vi "Actor Core.vi"(8 "error in":errorcluster, 11 "IMAQdx Actor in":refnum<class "IMAQdx Actor.lvclass">) -> (0 "error out":errorcluster, 3 "Actor out":refnum<class "Actor.lvclass">)   [LabVIEW 2020, in "IMAQdx Actor.lvlib" / "IMAQdx Actor.lvclass"]
doc: "(<B>Filename</B>: Actor Framework.lvlib:Actor.lvclass:Actor Core.vi)\n\nReceives messages to the actor, reacts to them, and initiates any error handling that may shut the actor down.\n\nDescendant classes may override this VI to append parallel tasks for the actor to complete while it handles messages. Overrides use the Call Parent Method node."
uses:
  IMAQdx Actor.lvclass
  C:/Users/AlexK/work/LabVIEW Programme/POLARIS-AS-3-Cams/Submodules/HIJ Vision/Camera Actors/Camera Actor/Camera Actor/Camera Actor.lvclass
  C:/Program Files (x86)/National Instruments/LabVIEW 2020/vi.lib/ActorFramework/Actor/Actor.lvclass
  <vilib>/ActorFramework/Actor/Actor.lvclass
  Camera Actor/Camera Actor/Operation Mode.ctl
  <vilib>/userdefined/High Color/IMAQdx.ctl
  <vilib>/vision/Image Controls.llb/IMAQ Image.ctl
  Camera Actor/Camera Actor/Camera Actor.lvclass/Camera Actor.ctl
  IMAQdx Actor.lvclass/IMAQdx Actor.ctl
  <vilib>/ActorFramework/Actor/Actor.lvclass/Actor.ctl
  <vilib>/ActorFramework/Message Enqueuer/Message Enqueuer.lvclass/Message Enqueuer.ctl
  Camera Actor/Camera Actor Messages/Publish Image Msg/Publish Image Msg.lvclass/Publish Image Msg.ctl
  <vilib>/ActorFramework/Report Error Msg/Report Error Msg.lvclass/Report Error Msg.ctl
  Camera Actor/Camera Actor/Write Image ref.vi
  <vilib>/ActorFramework/Message Enqueuer/Init from Existing Queue.vi
  <vilib>/ActorFramework/Message Enqueuer/Enqueue.vi
  Camera Actor/Camera Actor Messages/Publish Image Msg/Publish Image Msg.lvclass
  C:/Program Files (x86)/National Instruments/LabVIEW 2020/vi.lib/ActorFramework/Message/Message.lvclass
  <vilib>/ActorFramework/Report Error Msg/Report Error Msg.lvclass
  <vilib>/ActorFramework/Message Priority Queue/Priority Enqueue.vi
  Camera Actor/Camera Actor/Camera Actor.lvclass
  <vilib>/ActorFramework/Message Enqueuer/Message Enqueuer.lvclass
  <vilib>/vision/driver/NI_Vision_Acquisition_Software.lvlib
panel:
  in  "Image":T1
  in  "Session In":T2 caption="Session"
  in  "Mode":T3=enum."Stop"
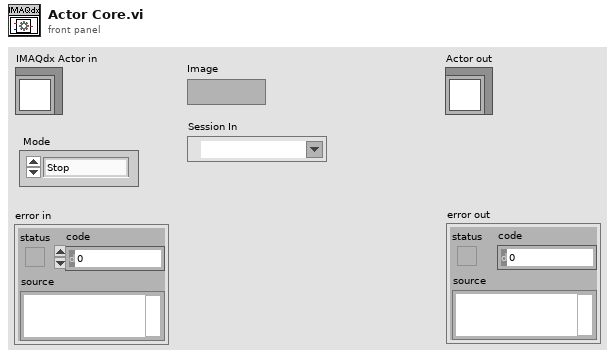
[diagram p1: front panel]
types:
  T1 = typedef "IMAQ Image.ctl" = refnum<image>
  T2 = typedef "IMAQdx.ctl" = refnum<k21>
  T3 = typedef "Camera Actor.lvlib/Camera Actor.lvclass/Operation Mode.ctl" = enum16{"Run", "Stop", "Exit", "Error", "Restart"}
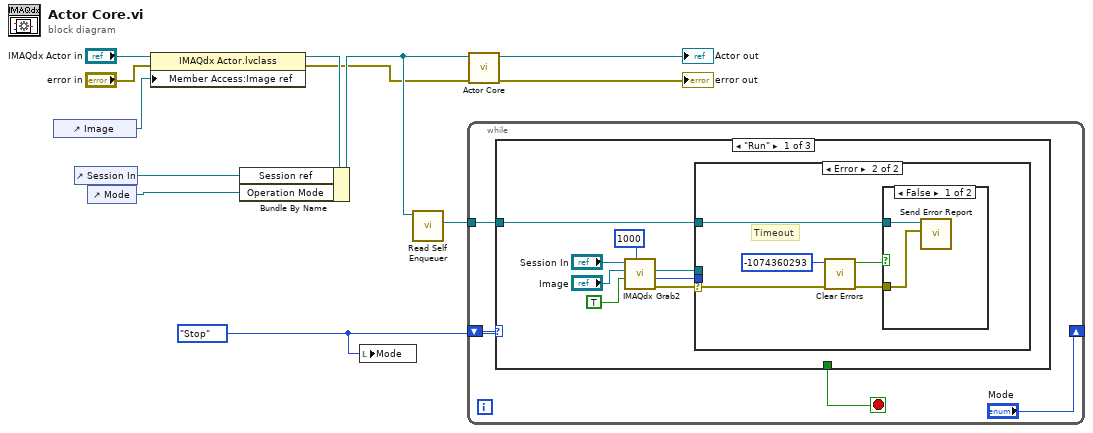
[diagram p0: block diagram]
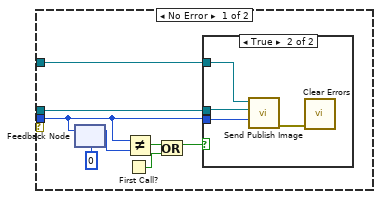
[diagram p2: hidden frame]
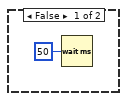
[diagram p3: hidden frame]
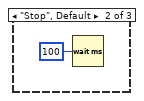
[diagram p5: hidden frame]
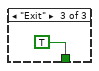
[diagram p6: hidden frame]
diagram:
  w7 = Operation_Mode."Stop" ("Operation Mode")
  n1 = control-ref of="Image"() -> (w3:refnum<vi>)
  n2 = control-ref of="Session In"() -> (w8:refnum<vi>)
  n3 = control-ref of="Mode"() -> (w9:refnum<vi>)
  n4 = property class="IMAQdx Actor.lvclass"(reference="IMAQdx Actor in", error in="error in", "Member Access:Image ref"=w3) -> (reference out=w4:refnum<class "IMAQdx Actor.lvclass">, error out=w1:errorcluster)
  n5 = Bundle By Name(cluster=w4, "Session ref"=w8, "Operation Mode"=w9) -> (w6:refnum<class "IMAQdx Actor.lvclass">)
  n6 = local write "Mode"(w7) -> ()
  n7 = call <vilib>:"Read Self Enqueuer.vi"("Actor"=w6) -> ("Self Enqueuer"=w5:refnum<class "Message Enqueuer.lvclass">)  [unwired: 10 in]
  n8 = while {
    shift-right: ["Mode"] -> _
    shift-left: w7 -> [w16]
    tunnel: w5 -> [w13]
    stop <- w15 stop-if-true
    n9 = case shown="\"Run\"" w16 {
      tunnel: [_ _ TRUE ("Value (Signaling)")] -> w15
      tunnel: w13 -> [w21 _ _]
      frame "Run" {
        n10 = call <vilib>:"IMAQdx Grab2.vi"("Timeout (ms)"=1000, "Wait for Next Buffer? (Yes)"=TRUE, "Image In"="Image", "Session In"="Session In") -> ("error out"=w19:errorcluster, "Buffer Number Out"=w20:u32, "Image Out"=w22:T1)  [unwired: 4 in, 1 out]
        n11 = case shown="Error" w19 {
          selector: w19 -> [_ w41]
          tunnel: w22 -> [w29 _]
          tunnel: w21 -> [w28 w42]
          tunnel: w20 -> [w27 _]
          frame No Error {
            n12 = feedback #1(u32 0 ("Buffer Number Out")) -> (w31:u32)
            n13 = feedback-in #1(w27) -> ()
            n14 = First Call?() -> (First Call?: T/F=w25:bool)
            n15 = Not Equal?(x=w27, y=w31) -> (x != y?=w30:bool)
            n16 = Or(x=w30, y=w25) -> (x .or. y?=w26:bool)
            n17 = case shown="True" w26 {
              tunnel: w29 -> [_ w34]
              tunnel: w28 -> [_ w37]
              tunnel: w27 -> [_ w36]
              frame False {
                n18 = Wait (ms)(milliseconds to wait=u32 50) -> ()  [unwired: 1 out]
              }
              frame True {
                n19 = call "Send Publish Image.vi"("Buffer Number"=w36, "Image"=w34, "Message Enqueuer"=w37) -> ("error out"=w35:errorcluster)  [unwired: 7 in, 1 out]
                n20 = call <vilib>:"Clear Errors.vi"("error in (no error)"=w35) -> ()  [unwired: 5 in, 2 out]
              }
            }
          }
          frame Error {
            # "Timeout"
            n21 = call <vilib>:"Clear Errors.vi"("error in (no error)"=w41, "specific error code to clear (0: all)"=-1074360293) -> ("error out"=w40:errorcluster, "specific error cleared?"=w38:bool)  [unwired: 4 in]
            n22 = case shown="False" w38 {
              tunnel: w42 -> [w44 _]
              tunnel: w40 -> [w43 _]
              frame False {
                n23 = call <vilib>:"Send Error Report.vi"("Error From Sender"=w43, "Message Enqueuer"=w44) -> ()  [unwired: 9 in, 1 out]
              }
              frame True {
              }
            }
          }
        }
      }
      frame "Stop", Default {
        n24 = Wait (ms)(milliseconds to wait=u32 100) -> ()  [unwired: 1 out]
      }
      frame "Exit" {
      }
    }
  }
  n25 = call-parent "Actor Core.vi"("error in"=w1, "Camera Actor in"=w6) -> ("error out"=→"error out":errorcluster, "Actor out"=→"Actor out":refnum<class "Actor.lvclass">)  [unwired: 8 in]
